vi "ReadCP_D.vi"(8 "error in (no error)":errorcluster, 10 "back to main":bool, 11 "VISA resource name":refnum<visa-resource-name>) -> (0 "error out":errorcluster, 1 "Supplementary Measurement":dbl, 2 "Capacitance Measurement":dbl, 3 "VISA resource name out":refnum<visa-resource-name>, 4 "Measurement Status":i32)   [LabVIEW 2016]
uses:
  global value.vi
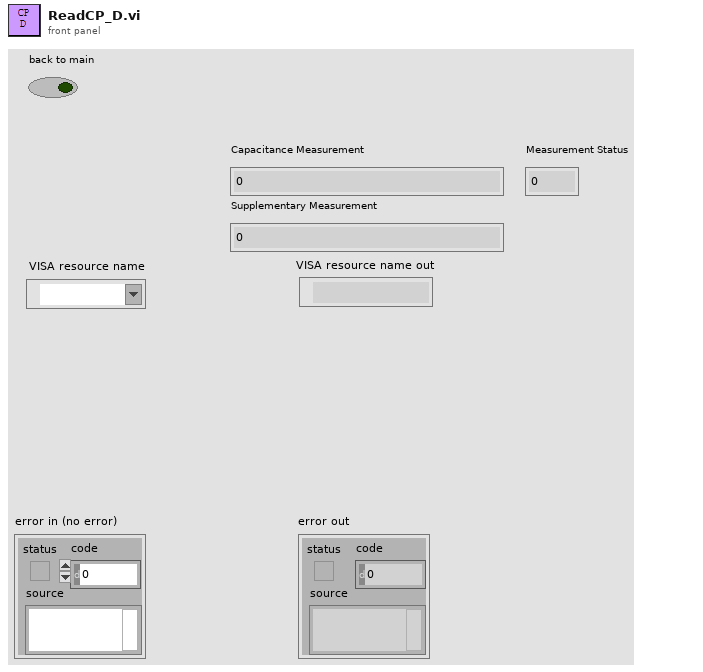
[diagram p1: front panel]
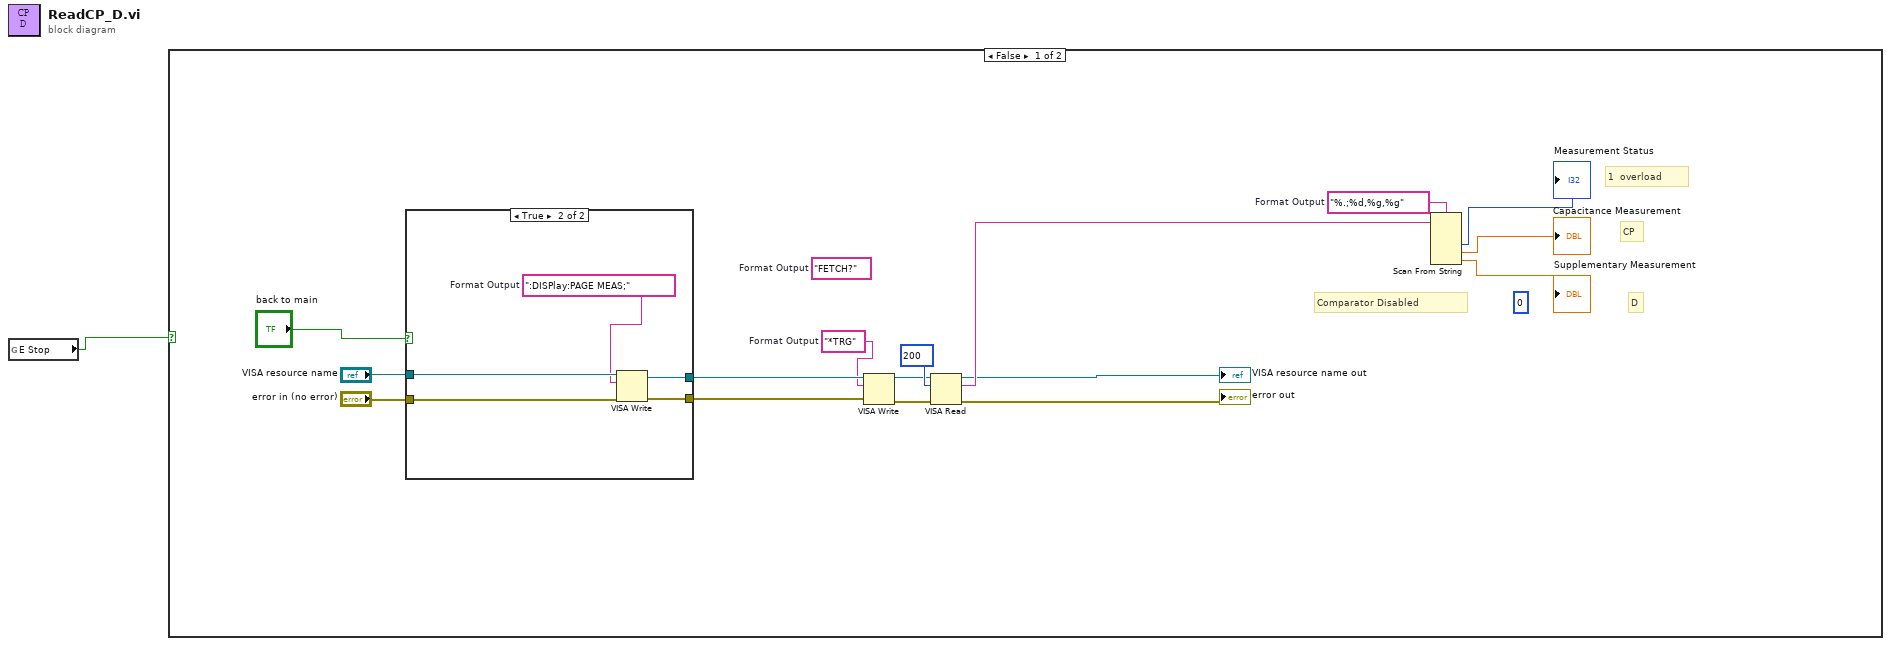
[diagram p0: block diagram]
diagram:
  n1 = global read "global value.vi" "E Stop"() -> (w1:bool)
  n2 = case shown="False" w1 {
    frame False {
      (unwired) "FETCH?"  # Format Output
      w3 = "*TRG"  # Format Output
      (unwired) 0
      w12 = "%.;%d,%g,%g"  # Format Output
      # "1  overload"
      # "Comparator Disabled"
      # "D"
      # "CP"
      n3 = case shown="True" "back to main" {
        tunnel: "VISA resource name" -> [w19 w24]
        tunnel: "error in (no error)" -> [w18 w23]
        tunnel: [w18 w22] -> w5
        tunnel: [w19 w21] -> w4
        frame False {
        }
        frame True {
          w20 = ":DISPlay:PAGE MEAS;"  # Format Output
          n4 = VISA Write(VISA resource name=w24, write buffer=w20, error in (no error)=w23) -> (VISA resource name out=w21:refnum<visa-resource-name>, error out=w22:errorcluster)  [unwired: 1 out]
        }
      }
      n5 = VISA Write(VISA resource name=w4, write buffer=w3, error in (no error)=w5) -> (VISA resource name out=w9:refnum<visa-resource-name>, error out=w8:errorcluster)  [unwired: 1 out]
      n6 = VISA Read(VISA resource name=w9, byte count=u32 200, error in (no error)=w8) -> (VISA resource name out=→"VISA resource name out":refnum<visa-resource-name>, read buffer=w16:string, error out=→"error out":errorcluster)  [unwired: 1 out]
      n7 = Scan From String(format string=w12, input string=w16) -> (output 1=→"Measurement Status":i32, output 2=→"Capacitance Measurement":dbl, output 3=→"Supplementary Measurement":dbl)  [unwired: 5 in, 3 out]
    }
    frame True {
    }
  }
